vi "FRCts20_WebMethods_WriteFormattedResponse.vi"(8 "error in (no error)":errorcluster, 10 "Response Cluster":variant, 11 "httpRequestID":u32) -> (0 "error out":errorcluster, 3 "httpRequestID out":u32)   [LabVIEW 2014]
doc: "Replaces the Write Reponse.vi to write a response specially formatted for the client."
uses:
  FRCts20_WebMethods.lvlib
  <vilib>/wsapi/NI_WebServices.lvlib
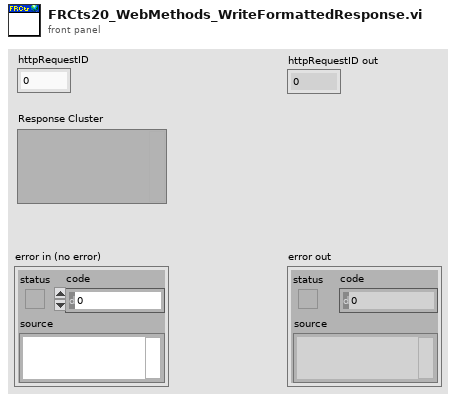
[diagram p1: front panel]
types:
  T1 = typedef "FRCts20_WebMethods.lvlib/FRCts20_WebMethods_ctl_returntype.ctl" = string
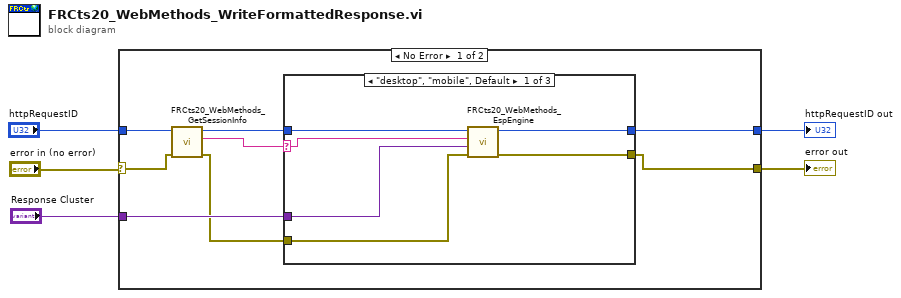
[diagram p0: block diagram]
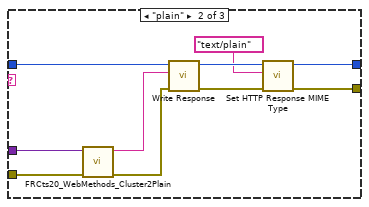
[diagram p2: hidden frame]
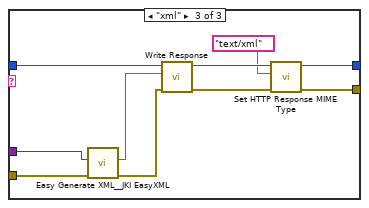
[diagram p3: hidden frame]
diagram:
  n1 = case shown="No Error" "error in (no error)" {
    selector: "error in (no error)" -> [w11 w41]
    tunnel: "httpRequestID" -> [w12 w40]
    tunnel: "Response Cluster" -> [w13 _]
    tunnel: [w6 w41] -> w3
    tunnel: [w7 w40] -> w2
    frame No Error {
      n2 = call "FRCts20_WebMethods_GetSessionInfo.vi"("error in"=w11, "httpRequestID"=w12) -> ("error out"=w10:errorcluster, "Return Type"=w9:T1, "httpRequestID out"=w8:u32)  [unwired: 7 in]
      n3 = case shown="\"desktop\", \"mobile\", Default" w9 {
        selector: w9 -> [w14 _ _]
        tunnel: w13 -> [w16 w22 w39]
        tunnel: w10 -> [w17 w23 w38]
        tunnel: w8 -> [w15 w29 w37]
        tunnel: [w19 w26 w31] -> w7
        tunnel: [w18 w25 w32] -> w6
        frame "desktop", "mobile", Default {
          n4 = call "FRCts20_WebMethods_EspEngine.vi"("error in (no error)"=w17, "Cluster"=w16, "Return Type"=w14, "httpRequestID"=w15) -> ("error out"=w18:errorcluster, "httpRequestID out"=w19:u32)  [unwired: 6 in]
        }
        frame "plain" {
          n5 = call "FRCts20_WebMethods_Cluster2Plain.vi"("error in (no error)"=w23, "Cluster"=w22) -> ("error out"=w24:errorcluster, "plain text"=w21:string)  [unwired: 8 in]
          n6 = call <vilib>:"Write Response.vi"("error in (no error)"=w24, "response string"=w21, "httpRequestID"=w29) -> ("error out"=w28:errorcluster, "httpRequestID out"=w27:u32)  [unwired: 7 in]
          n7 = call <vilib>:"Set HTTP Response MIME Type.vi"("error in (no error)"=w28, "MIME type (text/html)"="text/plain", "httpRequestID"=w27) -> ("error out"=w25:errorcluster, "httpRequestID out"=w26:u32)  [unwired: 7 in]
        }
        frame "xml" {
          n8 = call <vilib>:"Easy Generate XML__JKI EasyXML.vi"("error in (no error)"=w38, "LabVIEW Data"=w39) -> ("error out"=w36:errorcluster, "XML String"=w35:string)  [unwired: 8 in]
          n9 = call <vilib>:"Write Response.vi"("error in (no error)"=w36, "response string"=w35, "httpRequestID"=w37) -> ("error out"=w33:errorcluster, "httpRequestID out"=w34:u32)  [unwired: 7 in]
          n10 = call <vilib>:"Set HTTP Response MIME Type.vi"("error in (no error)"=w33, "MIME type (text/html)"="text/xml", "httpRequestID"=w34) -> ("error out"=w32:errorcluster, "httpRequestID out"=w31:u32)  [unwired: 7 in]
        }
      }
    }
    frame Error {
    }
  }
  "error out" <- w3
  "httpRequestID out" <- w2
